vi "testOnlineMap.vi"() -> ()   [LabVIEW 2011]
uses:
  <vilib>/vision/Image Controls.llb/IMAQ Image.ctl
  <vilib>/vision/NI_Vision_Development_Module.lvlib
  <vilib>/Analysis/NI_AALBase.lvlib
panel:
  in  "数组":string[](array[string])=["G8_E01B000.BLK", "G8_E01B001.BLK", "G8_E01B002.BLK", "G8_E01B003.BLK", "G8_E01B004.BLK", "G8_E01B005.BLK", "G8_E01B006.BLK", "G8_E01B007.BLK", "G8_E01B008.BLK", "G8_E01B009.BLK", "G8_E01B010.BLK", "G8_E01B011.BLK", "G8_E01B012.BLK", "G8_E01B013.BLK", "G8_E01B014.BLK", "G8_E01B015.BLK", "G8_E01B016.BLK", "G8_E01B017.BLK", "G8_E01B018.BLK"]
  in  "开始索引(0)":i32=386
  out "元素索引":i32
  out "Image":T1(plugin-control)
  out "数组 2":bool[](array[boolean])
  in  "DR/R parameter":T2={"frame_zero_0"=0, "frame_zero_1"=1, "frame_0"=3, "frame_1"=15}
  out "OnlineMap Array":T1[](array[typedef])
  in  "OnlineMap":cluster{"数组 1":i32[], "数组 2":i32[]}[](array[cluster])=[{"数组 1"=[2], "数组 2"=[6]}, {"数组 1"=[4], "数组 2"=[8]}, {"数组 1"=[2, 6], "数组 2"=[4, 8]}, {"数组 1"=[2, 4, 6, 8], "数组 2"=[0]}, {"数组 1"=[2, 4], "数组 2"=[6, 8]}]
  in  "DR/R array":T1[](array[typedef])
  out "datatype":u16(ring)=13 items=["U8"=11, "I16"=12, "U32"=13, "SGL"=14]
  out "FramesPerStim(100Hz)":i64=16
  out "FrameWidth":i64=704
  out "FrameHeight":i64=576
  in  "Blk目录":path=path "D:/Expt/test/run05_G4/E01"
  in  "stim ID":u8[](array[numeric])=[0, 2, 4, 6, 8]
  # "÷"
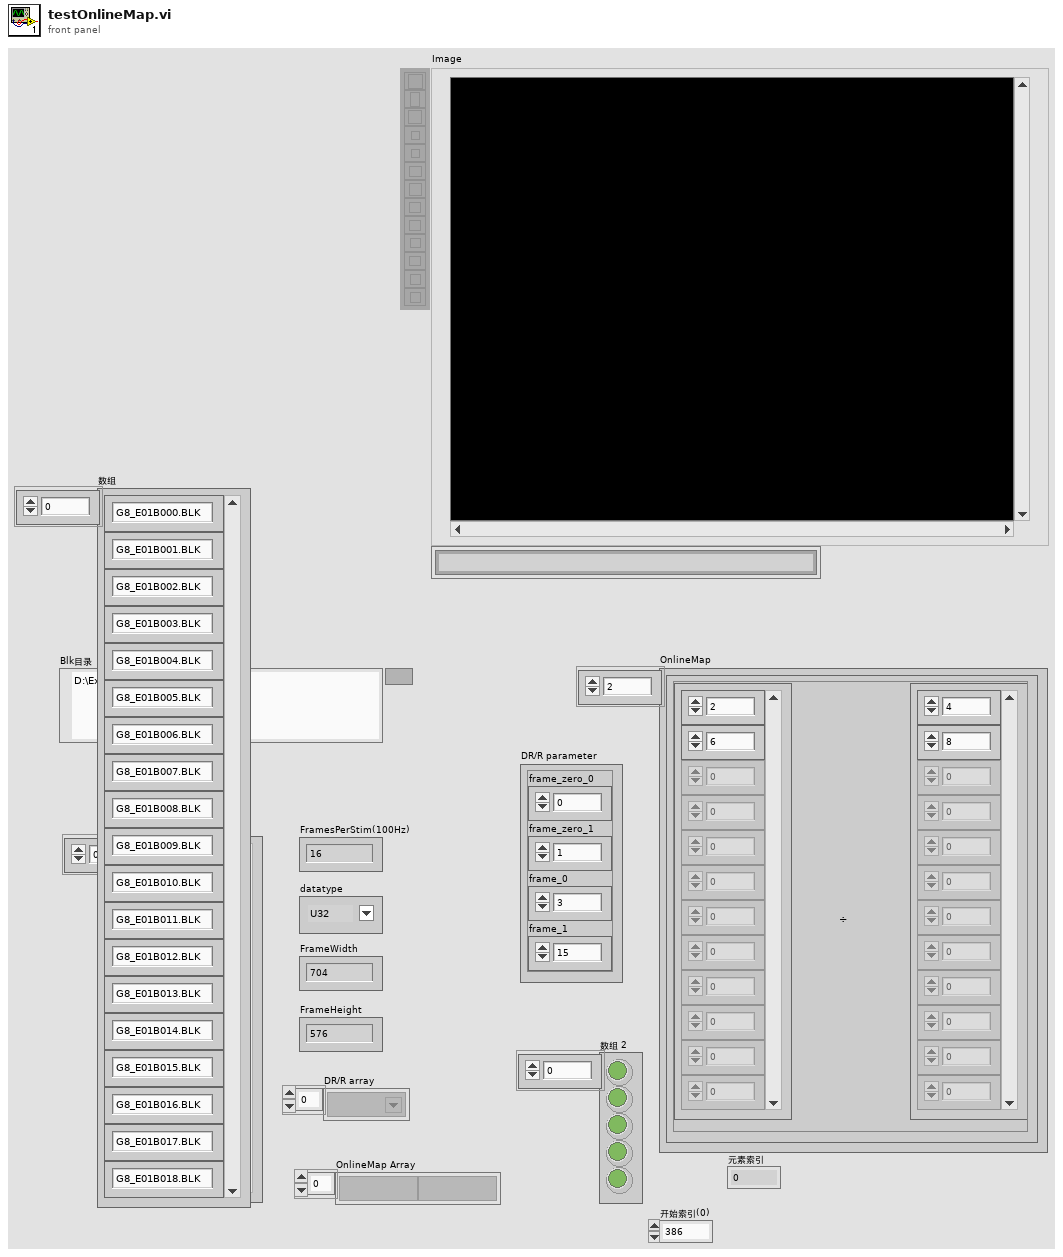
[diagram p1: front panel]
types:
  T1 = typedef "IMAQ Image.ctl" = refnum<image>
  T2 = cluster{"frame_zero_0":i32, "frame_zero_1":i32, "frame_0":i32, "frame_1":i32}
  T3 = typedef "Image Type" = u32
  T4 = enum16{"big-endian, network order", "native, host order", "little-endian"}
  T5 = cluster{"Mean Value":sgl, "Standard Variation":sgl, "Minimal Value":sgl, "Maximal Value":sgl, "Area (calibrated)":sgl, "Area (pixels)":u32, "%":sgl, "Calibration Valid":bool}
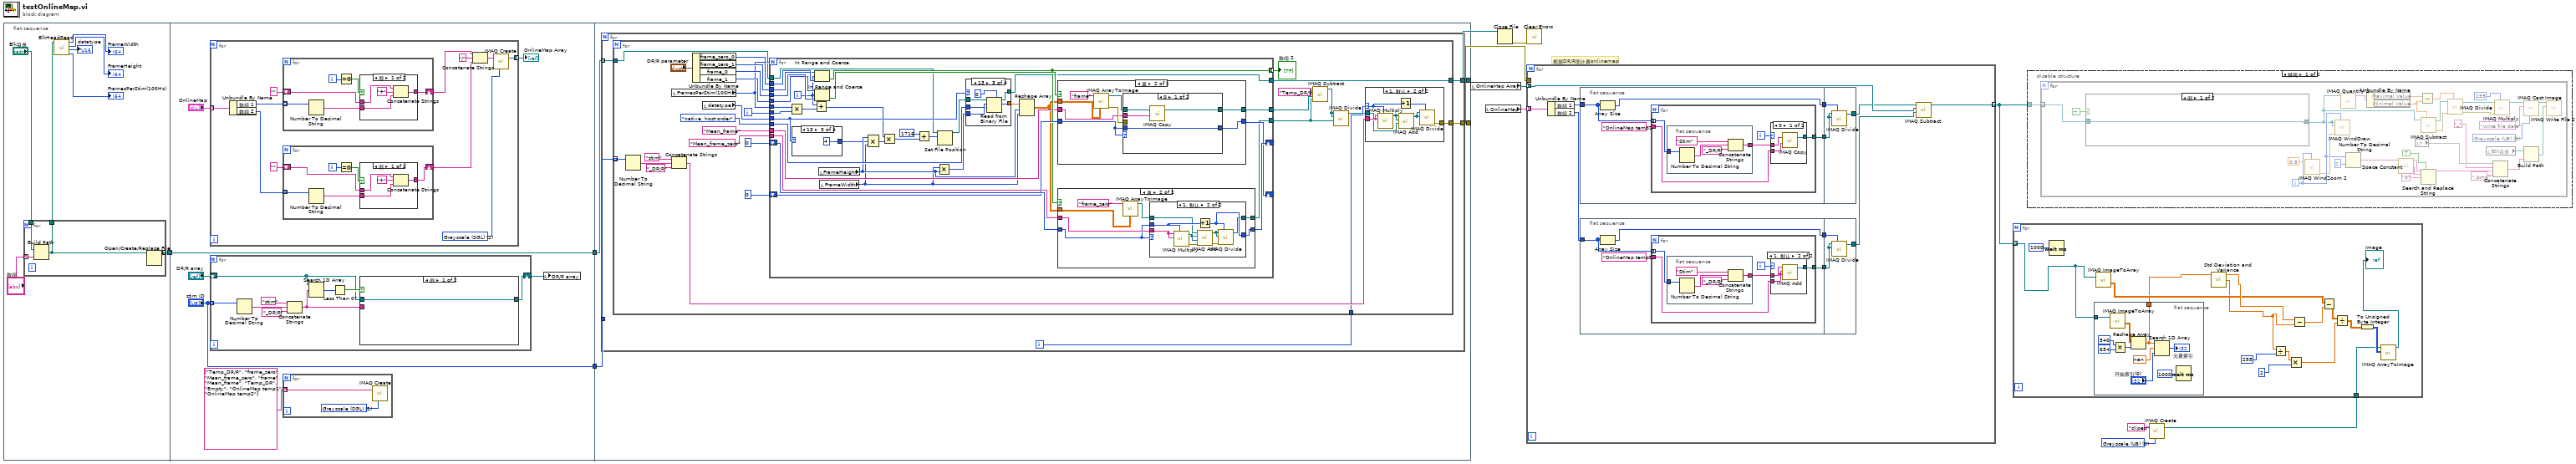
[diagram p0: block diagram]
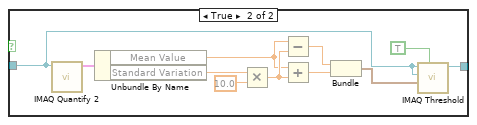
[diagram p2: hidden frame]
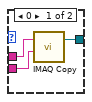
[diagram p4: hidden frame]
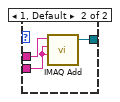
[diagram p5: hidden frame]
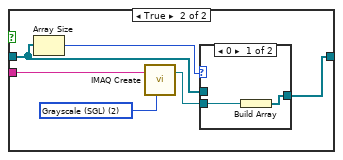
[diagram p8: hidden frame]
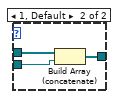
[diagram p9: hidden frame]
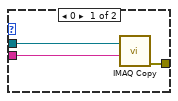
[diagram p10: hidden frame]
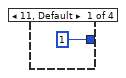
[diagram p11: hidden frame]
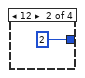
[diagram p12: hidden frame]
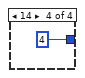
[diagram p13: hidden frame]
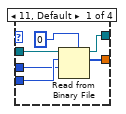
[diagram p14: hidden frame]
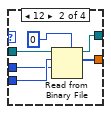
[diagram p15: hidden frame]
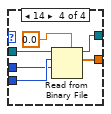
[diagram p16: hidden frame]
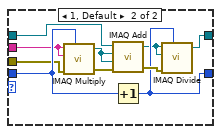
[diagram p18: hidden frame]
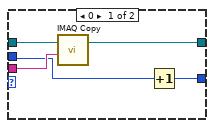
[diagram p20: hidden frame]
diagram:
  w2 = T3 0 items=["Grayscale (U8)", "Grayscale (I16)", "Grayscale (SGL)", "Complex (CSG)", "RGB (U32)", "HSL (U32)", "RGB (U64)", "Grayscale (U16)"] ("Image Type")
  # "根据DR/R图计算onlinemap"
  n1 = flat-sequence {
    tunnel: [w14] -> w7
    tunnel: ["stim ID"] -> w9
    tunnel: [w27] -> w8
    tunnel: w7 -> [w27]
    tunnel: [w91] -> w11
    tunnel: [w90] -> w10
    tunnel: w9 -> [w89]
    tunnel: w8 -> [w88]
    frame #0 {
      n2 = for {
        tunnel: "Blk目录" -> [w24]
        tunnel: [w23] -> w15
        tunnel: [w22] -> w14 mode=indexing
        tunnel: "数组" -> [w21] mode=indexing
        n3 = Build Path(base path=w24, name or relative path=w21) -> (appended path=w23:path)
        n4 = Open/Create/Replace File(file path (use dialog)=w23) -> (refnum out=w22:refnum<file>)  [unwired: 5 in, 2 out]
      }
      n5 = call "BlkHeadRead.vi"("BlkFilePath"=w15) -> ("FramesPerStim"=→"FramesPerStim(100Hz)":i32, "datatype"=→"datatype":i32, "FrameHeight"=→"FrameHeight":i32, "FrameWidth"=→"FrameWidth":i32)  [unwired: 5 in, 2 out]
    }
    frame #1 {
      n6 = for {
        tunnel: "OnlineMap" -> [w42] mode=indexing
        tunnel: [w32] -> w25 mode=indexing
        w40 = T3 2 items=["Grayscale (U8)", "Grayscale (I16)", "Grayscale (SGL)", "Complex (CSG)", "RGB (U32)", "HSL (U32)", "RGB (U64)", "Grayscale (U16)"] ("Image Type")
        n7 = Unbundle By Name(w42) -> ("数组 1"=w41:i32[], "数组 2"=w37:i32[])
        n8 = for {
          tunnel: w41 -> [w57] mode=indexing
          shift-right: [w55] -> w38
          shift-left: "" -> [w54]
          i -> [w59]
          n9 = Number To Decimal String(number=w57) -> (decimal integer string=w56:string)  [unwired: 1 in]
          n10 = Equal To 0?(x=w59) -> (x = 0?=w58:bool)
          n11 = case shown="假" w58 {
            tunnel: w56 -> [w60 w64]
            tunnel: [w63 w64] -> w55
            tunnel: w54 -> [w62 _]
            frame False {
              n12 = Concatenate Strings(w62, "+" ("字符串"), w60) -> (w63:string)
            }
            frame True {
            }
          }
        }
        n13 = for {
          tunnel: w37 -> [w46] mode=indexing
          shift-right: [w44] -> w35
          shift-left: "" -> [w43]
          i -> [w48]
          n14 = Number To Decimal String(number=w46) -> (decimal integer string=w45:string)  [unwired: 1 in]
          n15 = Equal To 0?(x=w48) -> (x = 0?=w47:bool)
          n16 = case shown="假" w47 {
            tunnel: w45 -> [w49 w53]
            tunnel: [w52 w53] -> w44
            tunnel: w43 -> [w51 _]
            frame False {
              n17 = Concatenate Strings(w51, "+" ("字符串"), w49) -> (w52:string)
            }
            frame True {
            }
          }
        }
        n18 = Concatenate Strings(w38, "/" ("字符串"), w35) -> (w33:string)
        n19 = call "IMAQ Create"("Image Name"=w33, "Image Type"=w40) -> ("New Image"=w32:T1)  [unwired: 3 in, 1 out]
      }
      "OnlineMap Array" <- w25
      n20 = for {
        tunnel: "stim ID" -> [w75] mode=indexing
        shift-right: [w67] -> w31
        shift-left: "DR/R array" -> [w68]
        n21 = Number To Decimal String(number=w75) -> (decimal integer string=w74:string)  [unwired: 1 in]
        n22 = Concatenate Strings("stim" ("字符串"), w74, "_DR/R" ("字符串")) -> (w69:string)
        n23 = Search 1D Array(1D array=w68, element=w69) -> (index of element=w71:i32)  [unwired: 1 in]
        n24 = Less Than 0?(x=w71) -> (x < 0?=w70:bool)
        n25 = case shown="假" w70 {
          tunnel: w69 -> [_ w82]
          tunnel: w68 -> [w76 w79]
          tunnel: [w76 w77] -> w67
          frame False {
          }
          frame True {
            w81 = T3 2 items=["Grayscale (U8)", "Grayscale (I16)", "Grayscale (SGL)", "Complex (CSG)", "RGB (U32)", "HSL (U32)", "RGB (U64)", "Grayscale (U16)"] ("Image Type")
            n26 = Array Size(array=w79) -> (size(s)=w80:i32)
            n27 = call "IMAQ Create"("Image Name"=w82, "Image Type"=w81) -> ("New Image"=w78:T1)  [unwired: 3 in, 1 out]
            n28 = case shown="0" w80 {
              tunnel: w79 -> [_ w87]
              tunnel: w78 -> [w84 w86]
              tunnel: [w83 w85] -> w77
              frame 0 {
                n29 = Build Array(w84) -> (w83:T1[])
              }
              frame 1, Default {
                n30 = Build Array (concatenate)(w87, w86) -> (w85:T1[])
              }
            }
          }
        }
      }
      n31 = for {
        tunnel: string[] ["Temp_DR/R", "frame_zero", "Mean_frame_zero", "frame", "Mean_frame", "Temp_DR", "Empty", "OnlineMap temp1", "OnlineMap temp2"] ("添加的数组") -> [w65] mode=indexing
        w66 = T3 2 items=["Grayscale (U8)", "Grayscale (I16)", "Grayscale (SGL)", "Complex (CSG)", "RGB (U32)", "HSL (U32)", "RGB (U64)", "Grayscale (U16)"] ("Image Type")
        n32 = call "IMAQ Create"("Image Name"=w65, "Image Type"=w66) -> ()  [unwired: 3 in, 2 out]
      }
      n33 = local write "DR/R array"(w31) -> ()
    }
    frame #2 {
      n34 = for {
        tunnel: [w96] -> w91
        tunnel: [w95] -> w90
        tunnel: w89 -> [w94]
        tunnel: w88 -> [w93] mode=indexing
        i -> [w92]
        n35 = for {
          tunnel: w94 -> [w103] mode=indexing
          tunnel: [w123] -> w96
          tunnel: [w109] -> w95
          tunnel: w93 -> [w101]
          tunnel: w92 -> [w97]
          i -> [w107]
          n36 = Number To Decimal String(number=w103) -> (decimal integer string=w106:string)  [unwired: 1 in]
          n37 = Concatenate Strings("stim" ("字符串"), w106, "_DR/R" ("字符串")) -> (w102:string)
          n38 = local read "FramesPerStim(100Hz)"() -> (w108:i64)
          n39 = Unbundle By Name("DR/R parameter") -> ("frame_zero_0"=w122:i32, "frame_zero_1"=w121:i32, "frame_0"=w119:i32, "frame_1"=w118:i32)
          n40 = local read "datatype"() -> (w110:u16)
          n41 = for {
            N: w108 -> [_]
            tunnel: w122 -> [w162]
            tunnel: w121 -> [w161]
            shift-right: [w167] -> _
            shift-left: 0 -> [w168]
            tunnel: w119 -> [w160]
            tunnel: w118 -> [w159]
            shift-right: [w165] -> _
            shift-left: 0 -> [w166]
            tunnel: [w163] -> w116 mode=indexing
            tunnel: "Mean_frame_zero" ("Image Name") -> [w157]
            tunnel: [w158] -> w100
            tunnel: "Mean_frame" ("Image Name") -> [w155]
            tunnel: [w156] -> w124
            tunnel: T4."native, host order" ("字节顺序(0:big-endian, network order)") -> [w153]
            tunnel: w110 -> [w150]
            tunnel: [w151] -> w109
            tunnel: w107 -> [w145]
            tunnel: w108 -> [w144]
            tunnel: w101 -> [w136]
            i -> [w142]
            n42 = Multiply(x=w144, y=w145) -> (x*y=w143:i64)
            n43 = case shown="13" w150 {
              tunnel: [i64 1 i64 2 i64 4 i64 4] -> w147
              frame 11, Default {
              }
              frame 12 {
              }
              frame 13 {
              }
              frame 14 {
              }
            }
            n44 = Add(x=w142, y=w143) -> (x+y=w141:i64)
            n45 = In Range and Coerce(upper limit=w161, x=w142, lower limit=w162) -> (In Range?=w163:bool)  [unwired: 1 out]
            n46 = In Range and Coerce(upper limit=w159, x=w142, lower limit=w160) -> (In Range?=w164:bool)  [unwired: 1 out]
            n47 = local read "FrameHeight"() -> (w148:i64)
            n48 = local read "FrameWidth"() -> (w146:i64)
            n49 = Compound Arithmetic op=MULTIPLY(w148, w147, w146) -> (w140:i64)
            n50 = Multiply(x=w141, y=w140) -> (x*y=w139:i64)
            n51 = Add(x=i64 1716, y=w139) -> (x+y=w137:i64)
            n52 = Multiply(x=w146, y=w148) -> (x*y=w149:i64)
            n53 = Set File Position(offset (in bytes) (0)=w137, refnum=w136) -> (refnum out=w154:refnum<file>)  [unwired: 2 in, 1 out]
            n54 = case shown="13" w150 {
              tunnel: w154 -> [w178 w183 w187 w195]
              tunnel: w149 -> [w177 w182 w189 w194]
              tunnel: w153 -> [w176 w181 w188 w193]
              tunnel: [w174 w180 w186 w192] -> w152
              tunnel: [w173 w179 w185 w191] -> w151
              frame 11, Default {
                n55 = Read from Binary File(5:u8 0, 9:w176, 10:w177, 11:w178) -> (2:w174:u8[], 3:w173:refnum<file>)  [unwired: 2 in, 2 out]
              }
              frame 12 {
                n56 = Read from Binary File(5:u16 0, 9:w181, 10:w182, 11:w183) -> (2:w180:u16[], 3:w179:refnum<file>)  [unwired: 2 in, 2 out]
              }
              frame 13 {
                n57 = Read from Binary File(5:u32 0, 9:w188, 10:w189, 11:w187) -> (2:w186:u32[], 3:w185:refnum<file>)  [unwired: 2 in, 2 out]
              }
              frame 14 {
                n58 = Read from Binary File(5:sgl 0.0, 9:w193, 10:w194, 11:w195) -> (2:w192:sgl[], 3:w191:refnum<file>)  [unwired: 2 in, 2 out]
              }
            }
            n59 = Reshape Array(w152, w148, w146) -> (w135:sgl[][])
            n60 = case shown="真" w164 {
              tunnel: w135 -> [_ w206]
              tunnel: w166 -> [w198 w199]
              tunnel: [w198 w202] -> w165
              tunnel: [w197 w201] -> w156
              tunnel: w155 -> [w197 w200]
              frame False {
              }
              frame True {
                n61 = call "IMAQ ArrayToImage"("Image Pixels (Float)"=w206, "Image"="frame" ("Image Name")) -> ("error out"=w203:errorcluster, "Image Out"=w204:T1)  [unwired: 8 in]
                n62 = case shown="0" w199 {
                  tunnel: w199 -> [w207 w220]
                  tunnel: w204 -> [w210 w219]
                  tunnel: w203 -> [_ w215]
                  tunnel: [w207 w214] -> w202
                  tunnel: [w208 w212] -> w201
                  tunnel: w200 -> [w209 w211]
                  frame 0 {
                    n63 = call "IMAQ Copy"("Image Dst"=w209, "Image Src"=w210) -> ("Image Dst Out"=w208:T1)  [unwired: 4 in, 1 out]
                  }
                  frame 1, Default {
                    n64 = call "IMAQ Multiply"("Image Src A"=w211, "Constant"=w220, "Image Dst"=w211, "error in (no error)"=w215) -> ("Image Dst Out"=w218:T1, "error out"=w216:errorcluster)  [unwired: 3 in]
                    n65 = call "IMAQ Add"("Image Src A"=w219, "Image Dst"=w218, "Image Src B"=w218, "error in (no error)"=w216) -> ("Image Dst Out"=w213:T1, "error out"=w217:errorcluster)  [unwired: 3 in]
                    n66 = Increment(x=w220) -> (x+1=w214:i32)
                    n67 = call "IMAQ Divide"("Image Src A"=w213, "Constant"=w214, "Image Dst"=w213, "error in (no error)"=w217) -> ("Image Dst Out"=w212:T1)  [unwired: 3 in, 1 out]
                  }
                }
              }
            }
            n68 = case shown="真" w163 {
              tunnel: w135 -> [_ w224]
              tunnel: w168 -> [w222 w226]
              tunnel: [w222 w229] -> w167
              tunnel: [w221 w228] -> w158
              tunnel: w157 -> [w221 w227]
              frame False {
              }
              frame True {
                n69 = call "IMAQ ArrayToImage"("Image Pixels (Float)"=w224, "Image"="frame_zero" ("Image Name")) -> ("Image Out"=w223:T1)  [unwired: 8 in, 1 out]
                n70 = case shown="1, 默认" w226 {
                  tunnel: w226 -> [w231 w243]
                  tunnel: [w230 w240] -> w229
                  tunnel: w223 -> [w234 w237]
                  tunnel: [w232 w236] -> w228
                  tunnel: w227 -> [w233 w235]
                  frame 0 {
                    n71 = call "IMAQ Copy"("Image Dst"=w233, "Image Src"=w234) -> ("Image Dst Out"=w232:T1)  [unwired: 4 in, 1 out]
                    n72 = Increment(x=w231) -> (x+1=w230:i32)
                  }
                  frame 1, Default {
                    n73 = call "IMAQ Multiply"("Image Src A"=w235, "Constant"=w243, "Image Dst"=w235) -> ("Image Dst Out"=w238:T1, "error out"=w241:errorcluster)  [unwired: 4 in]
                    n74 = Increment(x=w243) -> (x+1=w240:i32)
                    n75 = call "IMAQ Add"("Image Src A"=w237, "Image Dst"=w238, "Image Src B"=w238, "error in (no error)"=w241) -> ("Image Dst Out"=w239:T1, "error out"=w242:errorcluster)  [unwired: 3 in]
                    n76 = call "IMAQ Divide"("Image Src A"=w239, "Constant"=w240, "Image Dst"=w239, "error in (no error)"=w242) -> ("Image Dst Out"=w236:T1)  [unwired: 3 in, 1 out]
                  }
                }
              }
            }
          }
          "数组 2" <- w116
          n77 = call "IMAQ Subtract"("Image Src A"=w100, "Image Dst"="Temp_DR/R" ("Image Name"), "Image Src B"=w124) -> ("Image Dst Out"=w99:T1)  [unwired: 4 in, 1 out]
          n78 = call "IMAQ Divide"("Image Src A"=w99, "Image Dst"=w99, "Image Src B"=w100) -> ("Image Dst Out"=w98:T1)  [unwired: 4 in, 1 out]
          n79 = case shown="1, 默认" w97 {
            selector: w97 -> [_ w131]
            tunnel: w98 -> [w127 w132]
            tunnel: w102 -> [w126 w134]
            tunnel: [w125 w128] -> w123
            frame 0 {
              n80 = call "IMAQ Copy"("Image Dst"=w126, "Image Src"=w127) -> ("error out"=w125:errorcluster)  [unwired: 4 in, 1 out]
            }
            frame 1, Default {
              n81 = call "IMAQ Multiply"("Image Src A"=w134, "Constant"=w131, "Image Dst"=w134) -> ("Image Dst Out"=w133:T1)  [unwired: 4 in, 1 out]
              n82 = Increment(x=w131) -> (x+1=w130:i32)
              n83 = call "IMAQ Add"("Image Src A"=w133, "Image Dst"=w133, "Image Src B"=w132) -> ("Image Dst Out"=w129:T1)  [unwired: 4 in, 1 out]
              n84 = call "IMAQ Divide"("Image Src A"=w129, "Constant"=w130, "Image Dst"=w129) -> ("error out"=w128:errorcluster)  [unwired: 4 in, 1 out]
            }
          }
        }
      }
    }
  }
  n85 = local read "OnlineMap Array"() -> (w6:T1[])
  n86 = local read "OnlineMap"() -> (w5:cluster{"数组 1":i32[], "数组 2":i32[]}[])
  n87 = Close File(refnum=w10) -> (error out=w12:errorcluster)  [unwired: 1 in, 1 out]
  n88 = call <vilib>:"Clear Errors.vi"("error in (no error)"=w12) -> ()  [unwired: 6 in, 1 out]
  n89 = for {
    tunnel: w5 -> [w254] mode=indexing
    tunnel: w6 -> [w247] mode=indexing
    tunnel: [w244] -> w4 mode=indexing
    tunnel: w11 -> [_]
    n90 = Unbundle By Name(w254) -> ("数组 1"=w253:i32[], "数组 2"=w248:i32[])
    n91 = flat-sequence {
      tunnel: w253 -> [w280]
      tunnel: [w279] -> w252
      tunnel: [w278] -> w251
      tunnel: w252 -> [w299]
      tunnel: w251 -> [w300]
      tunnel: [w298] -> w246
      frame #0 {
        n92 = Array Size(array=w280) -> (size(s)=w278:i32)
        n93 = for {
          tunnel: w280 -> [w286] mode=indexing
          tunnel: "OnlineMap temp1" ("Image Name") -> [w284]
          tunnel: [w282] -> w279
          i -> [w283]
          n94 = flat-sequence {
            tunnel: w286 -> [w295]
            tunnel: [w293] -> w285
            frame #0 {
              n95 = Number To Decimal String(number=w295) -> (decimal integer string=w296:string)  [unwired: 1 in]
              n96 = Concatenate Strings("Stim", w296, "_DR/R" ("字符串")) -> (w293:string)
            }
          }
          n97 = case shown="0" w283 {
            tunnel: w285 -> [w289 w292]
            tunnel: w284 -> [w288 w291]
            tunnel: [w287 w290] -> w282
            frame 0 {
              n98 = call "IMAQ Copy"("Image Dst"=w288, "Image Src"=w289) -> ("Image Dst Out"=w287:T1)  [unwired: 4 in, 1 out]
            }
            frame 1, Default {
              n99 = call "IMAQ Add"("Image Src A"=w292, "Image Dst"=w291, "Image Src B"=w291) -> ("Image Dst Out"=w290:T1)  [unwired: 4 in, 1 out]
            }
          }
        }
      }
      frame #1 {
        n100 = call "IMAQ Divide"("Image Src A"=w299, "Constant"=w300, "Image Dst"=w299) -> ("Image Dst Out"=w298:T1)  [unwired: 4 in, 1 out]
      }
    }
    n101 = flat-sequence {
      tunnel: w248 -> [w257]
      tunnel: [w256] -> w250
      tunnel: [w255] -> w249
      tunnel: w250 -> [w276]
      tunnel: w249 -> [w277]
      tunnel: [w275] -> w245
      frame #0 {
        n102 = Array Size(array=w257) -> (size(s)=w255:i32)
        n103 = for {
          tunnel: w257 -> [w263] mode=indexing
          tunnel: "OnlineMap temp2" ("Image Name") -> [w261]
          tunnel: [w259] -> w256
          i -> [w260]
          n104 = flat-sequence {
            tunnel: w263 -> [w272]
            tunnel: [w270] -> w262
            frame #0 {
              n105 = Number To Decimal String(number=w272) -> (decimal integer string=w273:string)  [unwired: 1 in]
              n106 = Concatenate Strings("Stim", w273, "_DR/R" ("字符串")) -> (w270:string)
            }
          }
          n107 = case shown="1, 默认" w260 {
            tunnel: w262 -> [w266 w269]
            tunnel: w261 -> [w265 w268]
            tunnel: [w264 w267] -> w259
            frame 0 {
              n108 = call "IMAQ Copy"("Image Dst"=w265, "Image Src"=w266) -> ("Image Dst Out"=w264:T1)  [unwired: 4 in, 1 out]
            }
            frame 1, Default {
              n109 = call "IMAQ Add"("Image Src A"=w269, "Image Dst"=w268, "Image Src B"=w268) -> ("Image Dst Out"=w267:T1)  [unwired: 4 in, 1 out]
            }
          }
        }
      }
      frame #1 {
        n110 = call "IMAQ Divide"("Image Src A"=w276, "Constant"=w277, "Image Dst"=w276) -> ("Image Dst Out"=w275:T1)  [unwired: 4 in, 1 out]
      }
    }
    n111 = call "IMAQ Subtract"("Image Src A"=w246, "Image Dst"=w247, "Image Src B"=w245) -> ("Image Dst Out"=w244:T1)  [unwired: 4 in, 1 out]
  }
  n112 = disable-structure shown="禁用" {
    disable-tunnel: w4 -> [w301 _]
    frame Disabled {
      n113 = for {
        tunnel: w301 -> [w332] mode=indexing
        i -> [w330]
        w316 = T3 0 items=["Grayscale (U8)", "Grayscale (I16)", "Grayscale (SGL)", "Complex (CSG)", "RGB (U32)", "HSL (U32)", "RGB (U64)", "Grayscale (U16)"] ("Image Type")
        n114 = case shown="假" TRUE {
          tunnel: [w333 w338] -> w311
          tunnel: w332 -> [w333 w337]
          frame False {
          }
          frame True {
            n115 = call "IMAQ Quantify 2"("Image"=w337) -> ("Global Report"=w344:T5)  [unwired: 8 in, 2 out]
            n116 = Unbundle By Name(w344) -> ("Mean Value"=w336:sgl, "Standard Variation"=w335:sgl)
            n117 = Multiply(x=w335, y=sgl 10.0) -> (x*y=w342:sgl)
            n118 = Subtract(x=w336, y=w342) -> (x-y=w341:sgl)
            n119 = Add(x=w336, y=w342) -> (x+y=w340:sgl)
            n120 = Bundle(w341, w340) -> (w339:cluster{sgl, sgl})  [unwired: 1 in]
            n121 = call "IMAQ Threshold"("Keep/Replace Value (Replace)"=TRUE, "Range"=w339, "Image Dst"=w337, "Image Src"=w337) -> ("Image Dst Out"=w338:T1)  [unwired: 6 in, 1 out]
          }
        }
        n122 = call "IMAQ WindZoom 2"("Window Number (0...15)"=w330, "Zoom Factor"=sgl 0.5) -> ("error out"=w312:errorcluster)  [unwired: 6 in, 3 out]
        n123 = call "IMAQ WindDraw"("Window Number (0...15)"=w330, "error in (no error)"=w312, "Title"=w311, "Image"=w311) -> ()  [unwired: 6 in, 2 out]
        n124 = call "IMAQ Quantify 2"("Image"=w311) -> ("Global Report"=w314:T5)  [unwired: 8 in, 2 out]
        n125 = Number To Decimal String(number=w330, width (-)=i16 2 ("宽度(-)")) -> (decimal integer string=w326:string)
        n126 = Unbundle By Name(w314) -> ("Maximal Value"=w313:sgl, "Minimal Value"=w310:sgl)
        n127 = call <vilib>:"Space Constant.vi"() -> ("String"=w325:string)
        n128 = local read item#-1() -> (w328)
        n129 = Subtract(x=w313, y=w310) -> (x-y=w307:sgl)
        n130 = call "IMAQ Subtract"("Image Src A"=w311, "Constant"=w310) -> ("Image Dst Out"=w308:T1, "error out"=w309:errorcluster)  [unwired: 5 in]
        n131 = Search and Replace String(replace all?=TRUE ("替换全部？(F)"), input string=w326, search string=w325, replace string="0" ("替换字符串(\"\")")) -> (result string=w321:string)  [unwired: 4 in, 3 out]
        n132 = call "IMAQ Divide"("Image Src A"=w308, "Constant"=w307, "error in (no error)"=w309) -> ("Image Dst Out"=w305:T1, "error out"=w306:errorcluster)  [unwired: 4 in]
        n133 = local read "Blk目录"() -> (w319:path)
        n134 = Concatenate Strings(w328, "_" ("字符串"), w321, ".bmp" ("字符串")) -> (w318:string)
        n135 = call "IMAQ Multiply"("Image Src A"=w305, "Constant"=255, "error in (no error)"=w306) -> ("Image Dst Out"=w303:T1)  [unwired: 4 in, 1 out]
        n136 = call "IMAQ Cast Image"("Image Type"=w316, "Image Dst"="write file data" ("替换字符串(\"\")"), "Image Src"=w303) -> ("Image Dst Out"=w315:T1)  [unwired: 7 in, 1 out]
        n137 = Build Path(base path=w319, name or relative path=w318) -> (appended path=w317:path)
        n138 = call-poly "IMAQ Write File 2"("File Path"=w317, "Image"=w315) -> ()  [unwired: 8 in, 2 out]
      }
    }
    frame Enabled {
    }
  }
  n139 = call "IMAQ Create"("Image Name"="cliped", "Image Type"=w2) -> ("New Image"=w1:T1)  [unwired: 3 in, 1 out]
  n140 = for {
    tunnel: w4 -> [w359] mode=indexing
    tunnel: w1 -> [w348]
    n141 = Wait (ms)(milliseconds to wait=u32 1000 ("等待时间（毫秒）")) -> ()  [unwired: 1 out]
    n142 = flat-sequence {
      tunnel: w359 -> [w363]
      tunnel: [w361] -> w346
      frame #0 {
        n143 = call "IMAQ ImageToArray"("Image"=w363) -> ("Image Pixels (Float)"=w370:sgl[][])  [unwired: 3 in, 4 out]
        n144 = Multiply(x=540 ("维数大小"), y=654 ("维数大小")) -> (x*y=w364:i32)
        n145 = Reshape Array(w370, w364) -> (w361:sgl[])
        n146 = Search 1D Array(1D array=w361, element=nan ("standard deviation"), start index (0)="开始索引(0)") -> (index of element=→"元素索引":i32)
        n147 = Wait (ms)(milliseconds to wait=u32 1000 ("等待时间（毫秒）")) -> ()  [unwired: 1 out]
      }
    }
    n148 = call "IMAQ ImageToArray"("Image"=w359) -> ("Image Pixels (Float)"=w354:sgl[][])  [unwired: 3 in, 4 out]
    n149 = call <vilib>:"Std Deviation and Variance.vi"("X"=w346) -> ("mean"=w358:dbl, "standard deviation"=w345:dbl)  [unwired: 1 in, 1 out]
    n150 = Divide(x=w345, y=255) -> (x/y=w356:dbl)
    n151 = Multiply(x=w356, y=2) -> (x*y=w351:dbl)
    n152 = Subtract(x=w358, y=w345) -> (x-y=w353:dbl)
    n153 = Subtract(x=w354, y=w353) -> (x-y=w352:dbl[][])
    n154 = Divide(x=w352, y=w351) -> (x/y=w350:dbl[][])
    n155 = To Unsigned Byte Integer(number=w350) -> (unsigned 8bit integer=w349:u8[][])
    n156 = call "IMAQ ArrayToImage"("Image Pixels (U8)"=w349, "Image"=w348) -> ("Image Out"=→"Image":T1)  [unwired: 8 in, 1 out]
  }
